vi "调用.vi"   [LabVIEW 2017]
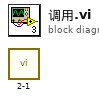
[diagram p0: block diagram]
diagram:
  n1 = call "2-1.vi"() -> ()  [unwired: 3 in, 1 out]
